vi "setUp.vi"(8 "error in (no error)":errorcluster, 11 "reference in":refnum<class "Test TCP Nested Endpoint.lvclass">) -> (0 "error out":errorcluster, 3 "reference out":refnum<class "Test TCP Nested Endpoint.lvclass">)   [LabVIEW 2020, in "Test TCP Nested Endpoint.lvclass"]
doc: "setUp runs prior to the test method during test execution. Use this method to initialize any object data required by your tests."
uses:
  Test TCP Nested Endpoint.lvclass
  <vilib>/addons/_JKI Toolkits/VI Tester/TestCase.llb/TestCase.lvclass
  <vilib>/ActorFramework/Actor/Actor.lvclass
  <vilib>/ActorFramework/Message Queue/Message Queue.lvclass
  Source/Protocols/TCP Strategy/TCP Stream Listener/TCP Stream Listener.lvclass
  Source/Protocols/TCP Strategy/TCP Stream Initiator/TCP Stream Initiator.lvclass
  Source/Protocols/TCP Strategy/TCP Stream/TCP Stream.lvclass
  Source/Ciphers/AES/AES.lvclass
  Source/Ciphers/AES/Ton Plomp Encryption/AES-Modes.ctl
  Source/Ciphers/AES/Ton Plomp Encryption/Encryption.lvlib
  Source/Nested Endpoint/Nested Endpoint/Nested Endpoint.lvclass
  Source/Network Endpoint/Network Endpoint/Network Endpoint.lvclass
  Source/Abstract Classes/Message Stream/Message Stream.lvclass
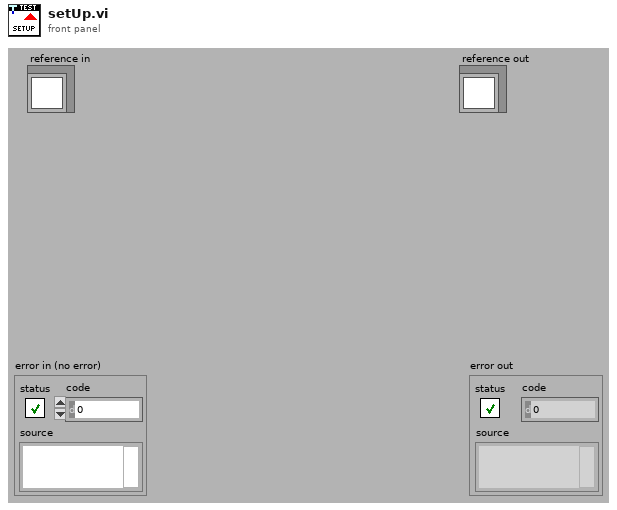
[diagram p1: front panel]
types:
  T1 = typedef "Encryption.lvlib/AES-Modes.ctl" = enum16{"ECB", "CBC", "CFB128", "OFB"}
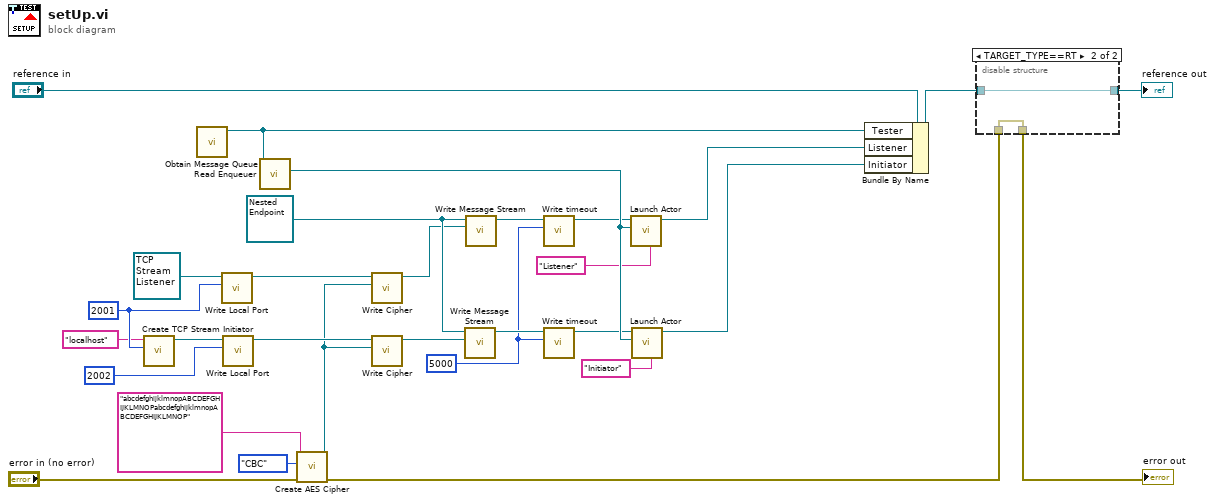
[diagram p0: block diagram]
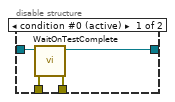
[diagram p2: hidden frame]
diagram:
  w3 = 5000 ("timeout")
  w23 = u16 2001 ("Port")
  w15 = refnum<class "Nested Endpoint.lvclass"> refnum ("Nested Endpoint.lvlib:Nested Endpoint.lvclass")
  n1 = call "Create TCP Stream Initiator.vi"("Remote Port"=w23, "Remote Address"="localhost" ("IP Address")) -> ("TCP Stream Initiator"=w25:refnum<class "TCP Stream Initiator.lvclass">)  [unwired: 9 in]
  n2 = call <vilib>:"Obtain Message Queue.vi"() -> ("Message Queue"=w9:refnum<class "Message Queue.lvclass">)  [unwired: 10 in, 1 out]
  n3 = call "Write Local Port.vi"("local port"=w23, "TCP Stream in"=refnum<class "TCP Stream Listener.lvclass"> refnum ("TCP Stream Listener.lvclass")) -> ("TCP Stream out"=w22:refnum<class "TCP Stream Listener.lvclass">)  [unwired: 9 in]
  n4 = call "Write Local Port.vi"("local port"=u16 2002, "TCP Stream in"=w25) -> ("TCP Stream out"=w21:refnum<class "TCP Stream Initiator.lvclass">)  [unwired: 9 in]
  n5 = call <vilib>:"Read Enqueuer.vi"("Message Queue"=w9) -> ("Message Enqueuer"=w26:refnum<class "Message Enqueuer.lvclass">)  [unwired: 10 in]
  n6 = call "Create AES Cipher.vi"("error in (no error)"="error in (no error)", "Operation Mode"=AES-Modes."CBC", "Cipher Key"="abcdefghijklmnopABCDEFGHIJKLMNOPabcdefghijklmnopABCDEFGHIJKLMNOP") -> ("error out"=w17:errorcluster, "AES out"=w16:refnum<class "AES.lvclass">)  [unwired: 7 in]
  n7 = call "Write Cipher.vi"("Cipher"=w16, "Message Stream in"=w22) -> ("Message Stream out"=w14:refnum<class "TCP Stream Listener.lvclass">)  [unwired: 9 in]
  n8 = call "Write Cipher.vi"("Cipher"=w16, "Message Stream in"=w21) -> ("Message Stream out"=w13:refnum<class "TCP Stream Initiator.lvclass">)  [unwired: 9 in]
  n9 = call "Write Message Stream.vi"("Message Stream"=w13, "Network Endpoint in"=w15) -> ("Network Endpoint out"=w5:refnum<class "Nested Endpoint.lvclass">)  [unwired: 9 in]
  n10 = call "Write Message Stream.vi"("Message Stream"=w14, "Network Endpoint in"=w15) -> ("Network Endpoint out"=w7:refnum<class "Nested Endpoint.lvclass">)  [unwired: 9 in]
  n11 = call "Write timeout.vi"("timeout"=w3, "Network Endpoint in"=w7) -> ("Network Endpoint out"=w6:refnum<class "Nested Endpoint.lvclass">)  [unwired: 9 in]
  n12 = call "Write timeout.vi"("timeout"=w3, "Network Endpoint in"=w5) -> ("Network Endpoint out"=w4:refnum<class "Nested Endpoint.lvclass">)  [unwired: 9 in]
  n13 = call <vilib>:"Launch Actor.vi"("Debug Alias"="Listener", "Actor-to-Caller Enqueuer"=w26, "Actor"=w6) -> ("Caller-To-Actor Enqueuer"=w11:refnum<class "Message Enqueuer.lvclass">)  [unwired: 7 in, 1 out]
  n14 = call <vilib>:"Launch Actor.vi"("Debug Alias"="Initiator", "Actor-to-Caller Enqueuer"=w26, "Actor"=w4) -> ("Caller-To-Actor Enqueuer"=w10:refnum<class "Message Enqueuer.lvclass">)  [unwired: 7 in, 1 out]
  n15 = Bundle By Name(cluster="reference in", "Tester"=w9, "Listener"=w11, "Initiator"=w10) -> (w27:refnum<class "Test TCP Nested Endpoint.lvclass">)
  n16 = disable-structure shown="TARGET_TYPE==RT" {
    disable-tunnel: w17 -> [w34 w35]
    disable-tunnel: [w33 w35] -> w30
    disable-tunnel: [w32 w36] -> w28
    disable-tunnel: w27 -> [w31 w36]
    frame condition #0 (active) {
      n17 = call <vilib>:"WaitOnTestComplete.vi"("error in (no error)"=w34, "TestCase in"=w31) -> ("error out"=w33:errorcluster, "TestCase out"=w32:refnum<class "Test TCP Nested Endpoint.lvclass">)  [unwired: 8 in]
    }
    frame condition #1 {
    }
  }
  "error out" <- w30
  "reference out" <- w28
